vi "solar_app SOLARini Read (DBL).vi"(5 "Write If Not Found? (T)":bool=TRUE, 6 "Comment (Create only)":string, 7 "Section (\"\"=solar)":string, 9 "Default Value (DBL)":dbl, 10 "Key":string) -> (1 "Value (DBL) out":dbl, 2 "Found?":bool)   [LabVIEW 2018]
doc: "This reads a double float configuration key from the solar.ini configuration file."
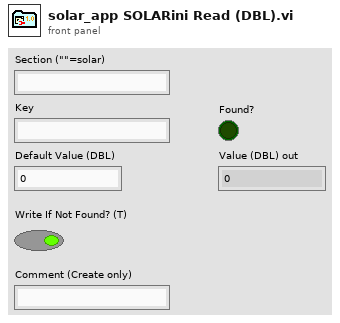
[diagram p1: front panel]
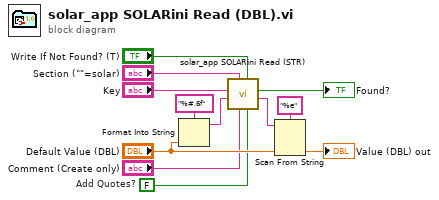
[diagram p0: block diagram]
diagram:
  w3 = FALSE  # Add Quotes?
  n1 = Format Into String(format string="%#.6f", "Default Value (DBL)") -> (resulting string=w4:string)  [unwired: 2 in, 1 out]
  n2 = call "solar_app SOLARini Read (STR).vi"("Add Quotes? (T)"=w3, "Write If Not Found? (T)"="Write If Not Found? (T)", "Comment (Create only)"="Comment (Create only)", "Section (\"\"=solar)"="Section (\"\"=solar)", "Default Value (STR)"=w4, "Key"="Key") -> ("Value (STR) out"=w10:string, "Found?"=→"Found?":bool)  [unwired: 4 in]
  n3 = Scan From String(format string="%e", input string=w10, default 1="Default Value (DBL)") -> (output 1=→"Value (DBL) out":dbl)  [unwired: 2 in, 3 out]
